vi "Check_Torque.vi"(11 "Torque":dbl) -> (3 "Pass/ Failure?":bool)   [LabVIEW 2019]
panel:
  # "13+-0.5 (kgf/cm)"
  # "8/1 эΘ10"
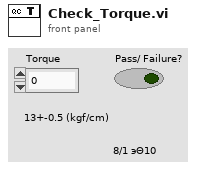
[diagram p1: front panel]
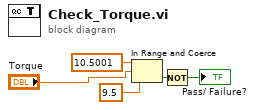
[diagram p0: block diagram]
diagram:
  n1 = In Range and Coerce(upper limit=10.5001, x="Torque", lower limit=9.5) -> (In Range?=w2:bool)  [unwired: 1 out]
  n2 = Not(x=w2) -> (.not. x?=→"Pass/ Failure?":bool)
